vi "KBoverRider.vi"(5 "1D array":T1(array[ring])) -> (2 "Cup up[T]":bool, 3 "CupWARD [Y]":bool, 4 "UP [U]":bool, 6 "IN [I]":bool, 8 "TOWERWARD [H]":bool, 10 "Down [J]":bool, 14 "RELEASE ALL":bool, 15 "OUT [K]":bool)   [LabVIEW 2011]
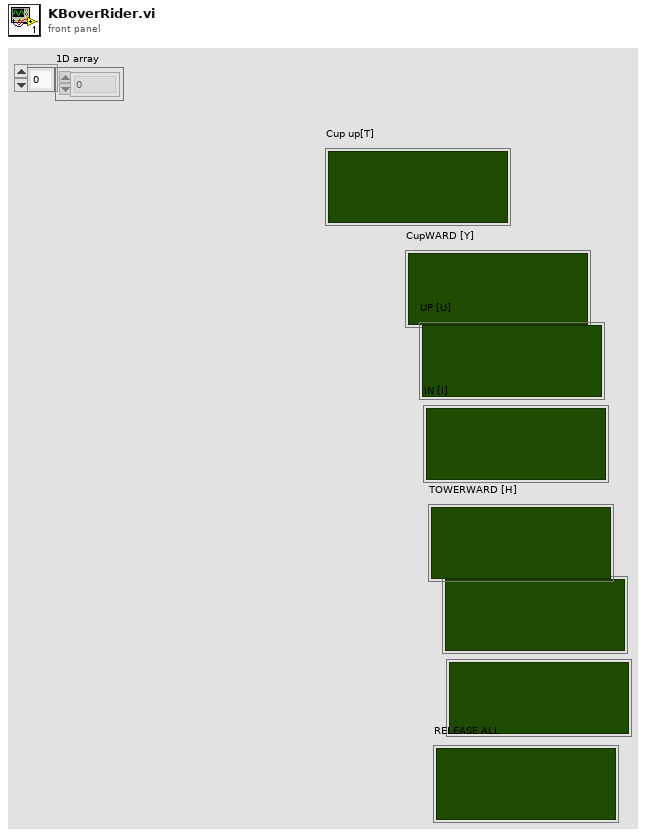
[diagram p1: front panel]
types:
  T1 = enum16{"0", "1", "2", "3", "4", "5", "6", "7", "8", "9", "A", "B", "C", "D", "E", "F", "G", "H", "I", "J", "K", "L", "M", "N", "O", "P", "Q", "R", "S", "T", "U", "V", "W", "X", "Y", "Z", "F1", "F2", "F3", "F4", "F5", "F6", "F7", "F8", "F9", "F10", "F11", "F12", "F13", "F14", "F15", "ADD", "BACK", "BACKSLASH", "CAPITAL", "COMMA", "DECIMAL", "DELETE", "DIVIDE", "DOWN", "END", "EQUALS", "ESCAPE", "GRAVE (`)", "HOME", "INSERT", "LBRACKET", "LCONTROL", "LEFT", "L ALT", "LSHIFT", "LWIN", "MINUS", "MULTIPLY", "NEXT", "NUMLOCK", "NUMPAD_0", "NUMPAD_1", "NUMPAD_2", "NUMPAD_3", "NUMPAD_4", "NUMPAD_5", "NUMPAD_6", "NUMPAD_7", "NUMPAD_8", "NUMPAD_9", "PAUSE", "PERIOD", "PRIOR (PG UP)", "RBRACKET", "RCONTROL", "RETURN", "RIGHT", "R ALT", "RSHIFT", "RWIN", "SCROLL", "SEMICOLON", "SLASH", "SPACE", "SUBTRACT", "TAB", "UP", "ENTER (num pad)", "' (quote)"}[]
  T2 = enum16{"0", "1", "2", "3", "4", "5", "6", "7", "8", "9", "A", "B", "C", "D", "E", "F", "G", "H", "I", "J", "K", "L", "M", "N", "O", "P", "Q", "R", "S", "T", "U", "V", "W", "X", "Y", "Z", "F1", "F2", "F3", "F4", "F5", "F6", "F7", "F8", "F9", "F10", "F11", "F12", "F13", "F14", "F15", "ADD", "BACK", "BACKSLASH", "CAPITAL", "COMMA", "DECIMAL", "DELETE", "DIVIDE", "DOWN", "END", "EQUALS", "ESCAPE", "GRAVE (`)", "HOME", "INSERT", "LBRACKET", "LCONTROL", "LEFT", "L ALT", "LSHIFT", "LWIN", "MINUS", "MULTIPLY", "NEXT", "NUMLOCK", "NUMPAD_0", "NUMPAD_1", "NUMPAD_2", "NUMPAD_3", "NUMPAD_4", "NUMPAD_5", "NUMPAD_6", "NUMPAD_7", "NUMPAD_8", "NUMPAD_9", "PAUSE", "PERIOD", "PRIOR (PG UP)", "RBRACKET", "RCONTROL", "RETURN", "RIGHT", "R ALT", "RSHIFT", "RWIN", "SCROLL", "SEMICOLON", "SLASH", "SPACE", "SUBTRACT", "TAB", "UP", "ENTER (num pad)", "' (quote)"}
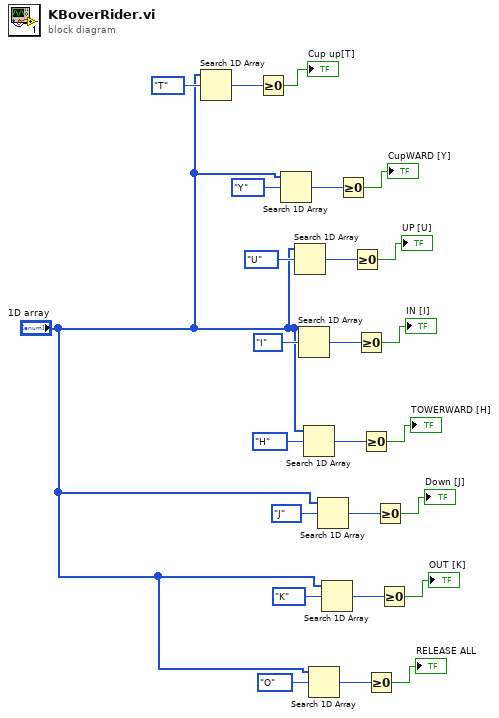
[diagram p0: block diagram]
diagram:
  n1 = Search 1D Array(1D array="1D array", element=T2."T" ("keys pressed[0]")) -> (index of element=w24:i32)  [unwired: 1 in]
  n2 = Greater Or Equal To 0?(x=w24) -> (x >= 0?=→"Cup up[T]":bool)
  n3 = Search 1D Array(1D array="1D array", element=T2."Y" ("keys pressed[0]")) -> (index of element=w22:i32)  [unwired: 1 in]
  n4 = Search 1D Array(1D array="1D array", element=T2."U" ("keys pressed[0]")) -> (index of element=w19:i32)  [unwired: 1 in]
  n5 = Search 1D Array(1D array="1D array", element=T2."I" ("keys pressed[0]")) -> (index of element=w15:i32)  [unwired: 1 in]
  n6 = Search 1D Array(1D array="1D array", element=T2."H" ("keys pressed[0]")) -> (index of element=w5:i32)  [unwired: 1 in]
  n7 = Search 1D Array(1D array="1D array", element=T2."O" ("keys pressed[0]")) -> (index of element=w3:i32)  [unwired: 1 in]
  n8 = Search 1D Array(1D array="1D array", element=T2."J" ("keys pressed[0]")) -> (index of element=w8:i32)  [unwired: 1 in]
  n9 = Search 1D Array(1D array="1D array", element=T2."K" ("keys pressed[0]")) -> (index of element=w12:i32)  [unwired: 1 in]
  n10 = Greater Or Equal To 0?(x=w22) -> (x >= 0?=→"CupWARD [Y]":bool)
  n11 = Greater Or Equal To 0?(x=w19) -> (x >= 0?=→"UP [U]":bool)
  n12 = Greater Or Equal To 0?(x=w15) -> (x >= 0?=→"IN [I]":bool)
  n13 = Greater Or Equal To 0?(x=w5) -> (x >= 0?=→"TOWERWARD [H]":bool)
  n14 = Greater Or Equal To 0?(x=w3) -> (x >= 0?=→"RELEASE ALL":bool)
  n15 = Greater Or Equal To 0?(x=w8) -> (x >= 0?=→"Down [J]":bool)
  n16 = Greater Or Equal To 0?(x=w12) -> (x >= 0?=→"OUT [K]":bool)
